vi "超标留样启动流程.vi"() -> ()   [LabVIEW 2016, in "科盛超标留样.lvlib"]
panel:
  in  "error in (no error)":errorcluster
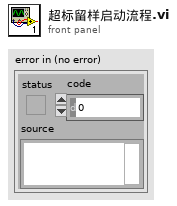
[diagram p1: front panel]
types:
  T1 = enum16{"触发采样", "触发采样完成", "供样命令", "供样完成", "留样命令", "留样完成"}
  T2 = cluster{"STEP":enum16{"open", "read", "write", "close"}, "写入缓冲区":string}
  T3 = cluster{"采样模式":enum16{"定时定量1", "定时定量2", "定流定量", "定时比例", "同步留样", "超标留样", "触发采样", "定时采样1", "定流供样", "定时采样2", "远程取样", "手动取样", "流量跟踪"}, "仪器状态":enum16{"待机", "运行中"}, "仪器时间":string, "瞬时流速(m3/s)":dbl, "当前COD值(mg/L)":dbl, "当前氨氮值(mg/L)":dbl, "当前温度(℃)":dbl, "开关量状态1":string, "开关量状态2":string, "开关量状态3":string, "A桶水样量(mL)":dbl, "B桶水样量(mL)":dbl}
  T4 = cluster{"采样泵1停0转":bool, "供样泵1停0转":bool, "泵1正转0反转":bool, "A桶搅拌1关0开":bool, "B桶搅拌1关0开":bool, "电控锁1关0开":bool, "流程1未完成0完成":bool, "外控泵1关0开":bool}
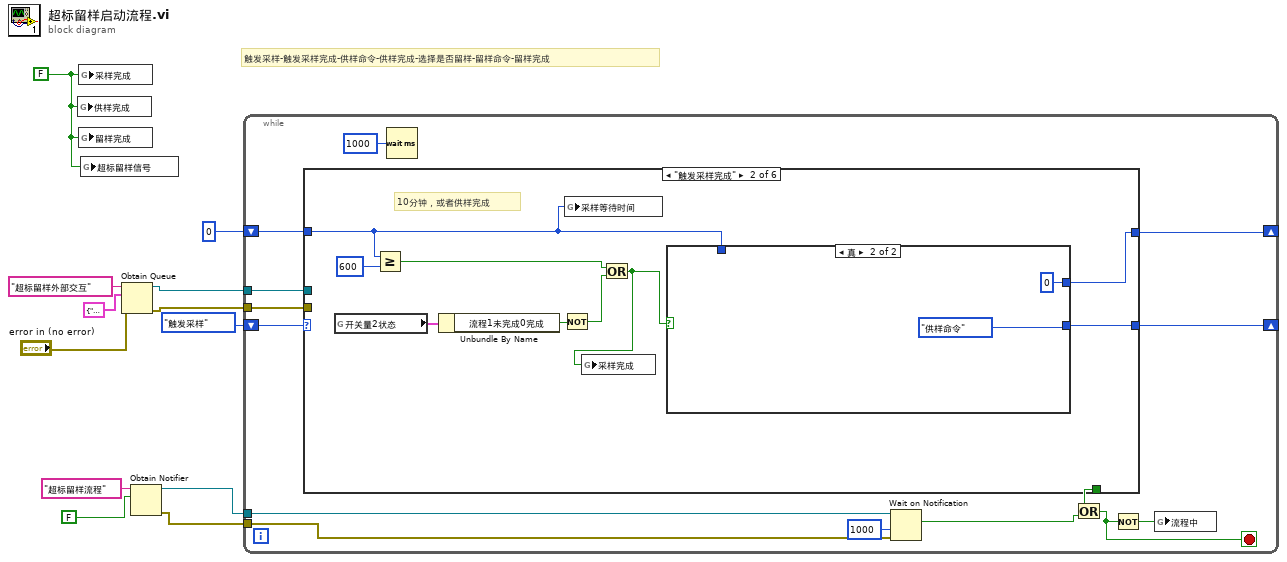
[diagram p0: block diagram]
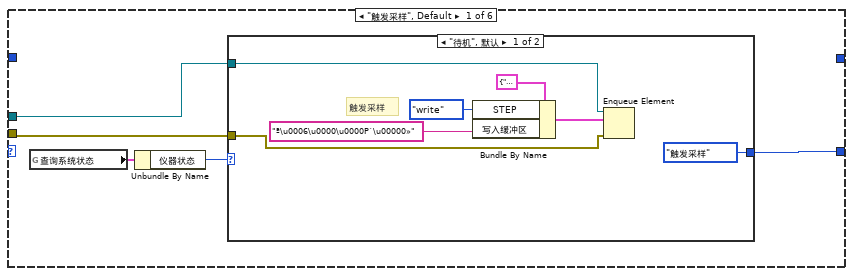
[diagram p2: hidden frame]
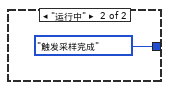
[diagram p3: hidden frame]
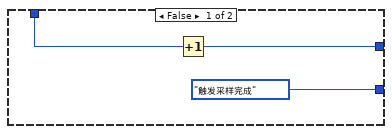
[diagram p4: hidden frame]
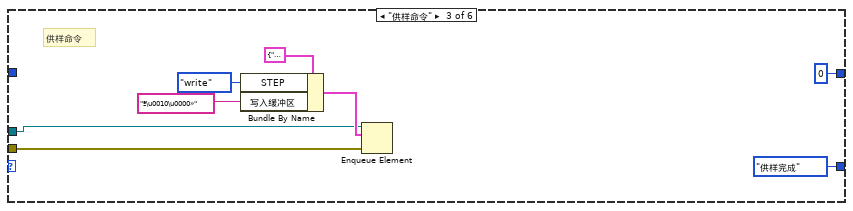
[diagram p5: hidden frame]
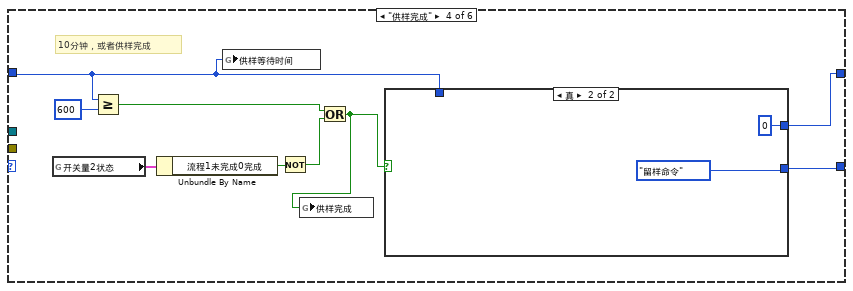
[diagram p6: hidden frame]
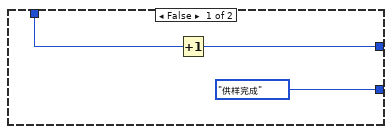
[diagram p7: hidden frame]
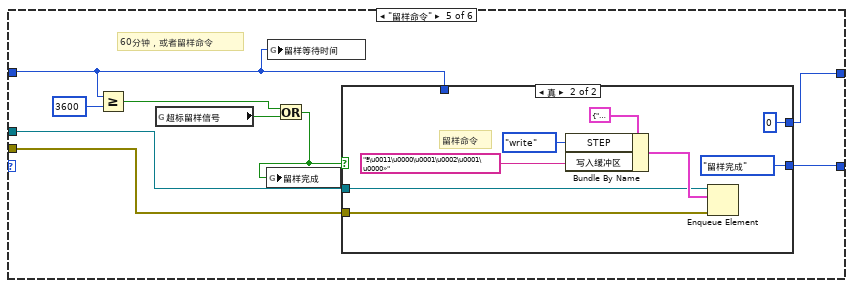
[diagram p8: hidden frame]
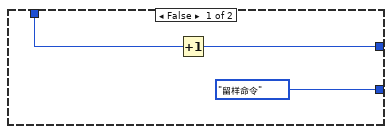
[diagram p9: hidden frame]
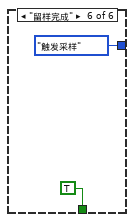
[diagram p10: hidden frame]
diagram:
  w1 = FALSE ("采样完成")
  # "触发采样-触发采样完成-供样命令-供样完成-选择是否留样-留样命令-留样完成"
  n1 = global write "超标留样全局.vi" "供样完成"(w1) -> ()
  n2 = global write "超标留样全局.vi" "采样完成"(w1) -> ()
  n3 = global write "超标留样全局.vi" "留样完成"(w1) -> ()
  n4 = global write "超标留样全局.vi" "超标留样信号"(w1) -> ()
  n5 = Obtain Queue(name (unnamed)="超标留样外部交互" ("名称（未命名）"), element data type=T2 {"STEP"=enum."write", "写入缓冲区"="ª\u0006\u0000\u0000P`\u00000»"}, error in (no error)="error in (no error)") -> (queue out=w8:refnum<queue>, error out=w7:errorcluster)  [unwired: 2 in, 1 out]
  n6 = Obtain Notifier(name (unnamed)="超标留样流程" ("名称（未命名）"), notification data type=FALSE ("采样完成")) -> (notifier out=w3:refnum<notifier>, error out=w2:errorcluster)  [unwired: 2 in, 1 out]
  n7 = while {
    shift-right: [w23] -> _
    shift-left: T1."触发采样" -> [w26]
    tunnel: w8 -> [w25]
    tunnel: w7 -> [w24]
    shift-right: [w20] -> _
    shift-left: 0 -> [w21]
    tunnel: w3 -> [w17]
    tunnel: w2 -> [w16]
    stop <- w14 stop-if-true
    n8 = case shown="\"触发采样完成\"" w26 {
      tunnel: w25 -> [w29 _ w57 _ w81 _]
      tunnel: w24 -> [w28 _ w56 _ w80 _]
      tunnel: [w27 w43 T1."供样完成" w63 w79 T1."触发采样"] -> w23
      tunnel: w21 -> [_ w40 _ w62 w76 _]
      tunnel: [_ w42 0 w64 w78 _] -> w20
      tunnel: [_ _ _ _ _ TRUE] -> w18
      frame "触发采样", Default {
        n9 = global read "超标留样全局.vi" "查询系统状态"() -> (w30:T3)
        n10 = Unbundle By Name(w30) -> ("仪器状态"=w31:enum16{"待机", "运行中"})
        n11 = case shown="\"待机\", 默认" w31 {
          tunnel: w29 -> [w34 _]
          tunnel: w28 -> [w33 _]
          tunnel: [T1."触发采样" T1."触发采样完成"] -> w27
          frame "待机", Default {
            # "触发采样"
            n12 = Bundle By Name(cluster=T2 {"STEP"=enum."open", "写入缓冲区"=""} ("元素"), "STEP"=enum16{"open", "read", "write", "close"}."write", "写入缓冲区"="ª\u0006\u0000\u0000P`\u00000»") -> (w37:T2)
            n13 = Enqueue Element(queue=w34, element=w37, error in (no error)=w33) -> ()  [unwired: 1 in, 3 out]
          }
          frame "运行中" {
          }
        }
      }
      frame "触发采样完成" {
        # "10分钟，或者供样完成"
        n14 = global read "超标留样全局.vi" "开关量2状态"() -> (w47:T4)
        n15 = Greater Or Equal?(x=w40, y=600) -> (x >= y?=w46:bool)
        n16 = Unbundle By Name(w47) -> ("流程1未完成0完成"=w45:bool)
        n17 = Not(x=w45) -> (.not. x?=w44:bool)
        n18 = global write "超标留样全局.vi" "采样等待时间"(w40) -> ()
        n19 = Or(x=w46, y=w44) -> (x .or. y?=w41:bool)
        n20 = global write "超标留样全局.vi" "采样完成"(w41) -> ()
        n21 = case shown="真" w41 {
          tunnel: [T1."触发采样完成" T1."供样命令"] -> w43
          tunnel: w40 -> [w50 _]
          tunnel: [w49 0] -> w42
          frame False {
            n22 = Increment(x=w50) -> (x+1=w49:i32)
          }
          frame True {
          }
        }
      }
      frame "供样命令" {
        # "供样命令"
        n23 = Bundle By Name(cluster=T2 {"STEP"=enum."open", "写入缓冲区"=""} ("元素"), "STEP"=enum16{"open", "read", "write", "close"}."write", "写入缓冲区"="ª\u0010\u0000»") -> (w60:T2)
        n24 = Enqueue Element(queue=w57, element=w60, error in (no error)=w56) -> ()  [unwired: 1 in, 3 out]
      }
      frame "供样完成" {
        # "10分钟，或者供样完成"
        n25 = global read "超标留样全局.vi" "开关量2状态"() -> (w69:T4)
        n26 = Greater Or Equal?(x=w62, y=600) -> (x >= y?=w68:bool)
        n27 = Unbundle By Name(w69) -> ("流程1未完成0完成"=w67:bool)
        n28 = global write "超标留样全局.vi" "供样等待时间"(w62) -> ()
        n29 = Not(x=w67) -> (.not. x?=w66:bool)
        n30 = Or(x=w68, y=w66) -> (x .or. y?=w65:bool)
        n31 = global write "超标留样全局.vi" "供样完成"(w65) -> ()
        n32 = case shown="真" w65 {
          tunnel: [T1."供样完成" T1."留样命令"] -> w63
          tunnel: w62 -> [w72 _]
          tunnel: [w71 0] -> w64
          frame False {
            n33 = Increment(x=w72) -> (x+1=w71:i32)
          }
          frame True {
          }
        }
      }
      frame "留样命令" {
        # "60分钟，或者留样命令"
        n34 = Greater Or Equal?(x=w76, y=3600) -> (x >= y?=w83:bool)
        n35 = global read "超标留样全局.vi" "超标留样信号"() -> (w82:bool)
        n36 = global write "超标留样全局.vi" "留样等待时间"(w76) -> ()
        n37 = Or(x=w83, y=w82) -> (x .or. y?=w77:bool)
        n38 = global write "超标留样全局.vi" "留样完成"(w77) -> ()
        n39 = case shown="真" w77 {
          tunnel: [T1."留样命令" T1."留样完成"] -> w79
          tunnel: w76 -> [w86 _]
          tunnel: [w85 0] -> w78
          tunnel: w81 -> [_ w89]
          tunnel: w80 -> [_ w88]
          frame False {
            n40 = Increment(x=w86) -> (x+1=w85:i32)
          }
          frame True {
            # "留样命令"
            n41 = Bundle By Name(cluster=T2 {"STEP"=enum."open", "写入缓冲区"=""} ("元素"), "STEP"=enum16{"open", "read", "write", "close"}."write", "写入缓冲区"="ª\u0011\u0000\u0001\u0002\u0001\u0000»") -> (w91:T2)
            n42 = Enqueue Element(queue=w89, element=w91, error in (no error)=w88) -> ()  [unwired: 1 in, 3 out]
          }
        }
      }
      frame "留样完成" {
      }
    }
    n43 = Wait (ms)(milliseconds to wait=u32 1000 ("等待时间（毫秒）")) -> ()  [unwired: 1 out]
    n44 = Wait on Notification(notifier=w17, timeout in ms (-1)=1000 ("超时毫秒(-1)"), error in (no error)=w16) -> (notification=w13:bool)  [unwired: 1 in, 3 out]
    n45 = Or(x=w18, y=w13) -> (x .or. y?=w14:bool)
    n46 = Not(x=w14) -> (.not. x?=w19:bool)
    n47 = global write "超标留样全局.vi" "流程中"(w19) -> ()
  }
